vi "Subsystem Sequencer Controller.vi"(8 "error in":errorcluster) -> ()   [LabVIEW 2018]
doc: "This VI executes continuously carrying out the current operation and responding to updates or new operations. It will often contain the timing or control code that is difficult to place directly in TeleOp. This VI generally opens all sensors and motors and isolates the rest of the robot code from knowing how the operations are carried out."
uses:
  <vilib>/Rock Robotics/WPI/Framework/Completion Status.ctl
  Subsystem Sequencer Setpoints.ctl
  Subsystem Sequencer Operations.ctl
  All Commands.ctl
  <vilib>/Rock Robotics/WPI/Solenoid/WPI_SolenoidValue.ctl
  <vilib>/Rock Robotics/WPI/Solenoid/WPI_SolenoidSetEnum.vi
  Wrist/Implementation/Wrist Published Globals.vi
panel:
  in  "In Position":dbl=90.0 format="%#_13g"
  in  "Pickup Position":dbl=-7.0 format="%#_13g"
  out "Value":dbl
  out "Cmd":T1
  in  "Interactive Values":T2
  out "Current\nCmd":string
  in  "Buttons":cluster{"Execute Cmd":bool, "Abort Cmd":bool}
  out "Command Timing":cluster{"Start Time (ms)":u32, "Iterations":i32}
  out "Status":T4
  # "Interactive Command: You may fill in the settings for a command\nand schedule it with the Execute button. You can observe and abort\nany command while fine tuning the code for the controller."
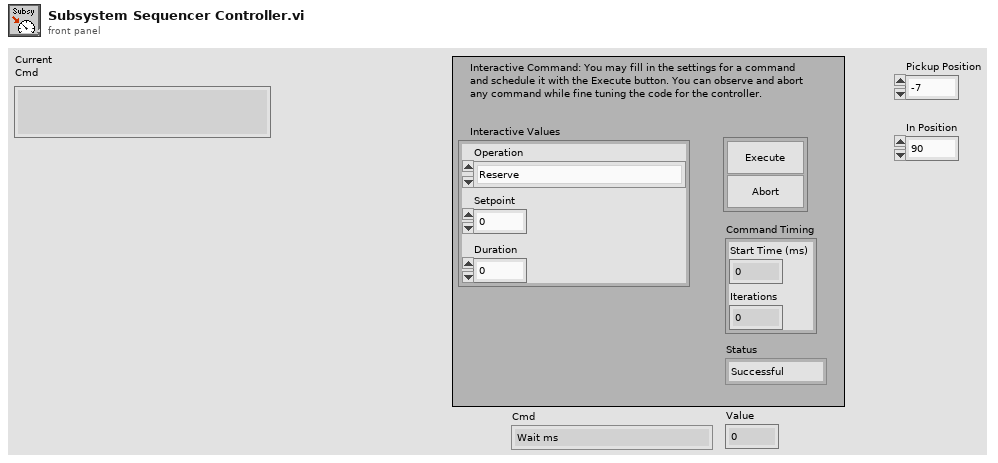
[diagram p1: front panel]
types:
  T1 = typedef "All Commands.ctl" = enum16{"Wait ms", "Drive - Stop Driving", "Drive - Drive Distance Straight", "Elevator - Elevator Stop", "Elevator - Elevator Set Position Wait", "Elevator - Elevator Set Position Start", "Elevator - Wait for Down Fast", "Wrist - Up", "Wrist - Down", "Wrist - Set Position", "Beak - Extend", "Beak - Retract", "Beak - Open", "Beak - Close", "Roller - Off", "Roller - Out", "Roller - In", "Roller - Set Position", "Roller - Wait for Cargo", "Drive - Set Power Straight", "Elevator - Wait Until Stopped", "Leg  - Piston Engage", "Wrist - Set Position Override"}
  T2 = typedef "Subsystem Sequencer Setpoints.ctl" = cluster{"Operation":T3, "Setpoint":dbl, "Duration":dbl}
  T3 = typedef "Subsystem Sequencer Operations.ctl" = enum16{"Reserve", "Read Current", "Run Sequence"}
  T4 = typedef "Completion Status.ctl" = enum16{"Successful", "Aborted", "Incomplete"}
  T5 = typedef "Command Status Info.ctl" = cluster{"Name":string, "Status":T4, "notifier out":T6}
  T6 = typedef "Completion Notifier.ctl" = refnum<notifier>
  T7 = cluster{"Current Command":T2, "Command Timing":cluster{"Start Time (ms)":u32, "Iterations":i32}, "Command Arguments":cluster{"Command Info":T5, "Description":string, "Default Command":T2, "queue out":refnum<queue>, "Subsystem Name":string}}
  T8 = typedef "WPI_SolenoidValue.ctl" = enum16{"Off", "On", "Forward", "Reverse"}
  T9 = typedef "Sequencer Type.ctl" = cluster{"Cmd":T1, "Value":dbl}
  T10 = typedef "WPI_SolenoidDevRef.ctl" = cluster{"DevStatus":errorcluster, "Pneumatics Control Module":u8, "Forward Solenoid Channel":T11, "Reverse Solenoid Channel":T11}
  T11 = typedef "WPI_SolenoidChannel.ctl" = enum8{"Solenoid 0", "Solenoid 1", "Solenoid 2", "Solenoid 3", "Solenoid 4", "Solenoid 5", "Solenoid 6", "Solenoid 7", "Invalid"}
  T12 = typedef "Elevator Telemetry.ctl" = cluster{"Is Moving?":bool, "Setpoint":dbl, "Velocity":dbl, "Position":dbl, "Top Limit":bool, "Bottom Limit":bool, "Applied Output":dbl}
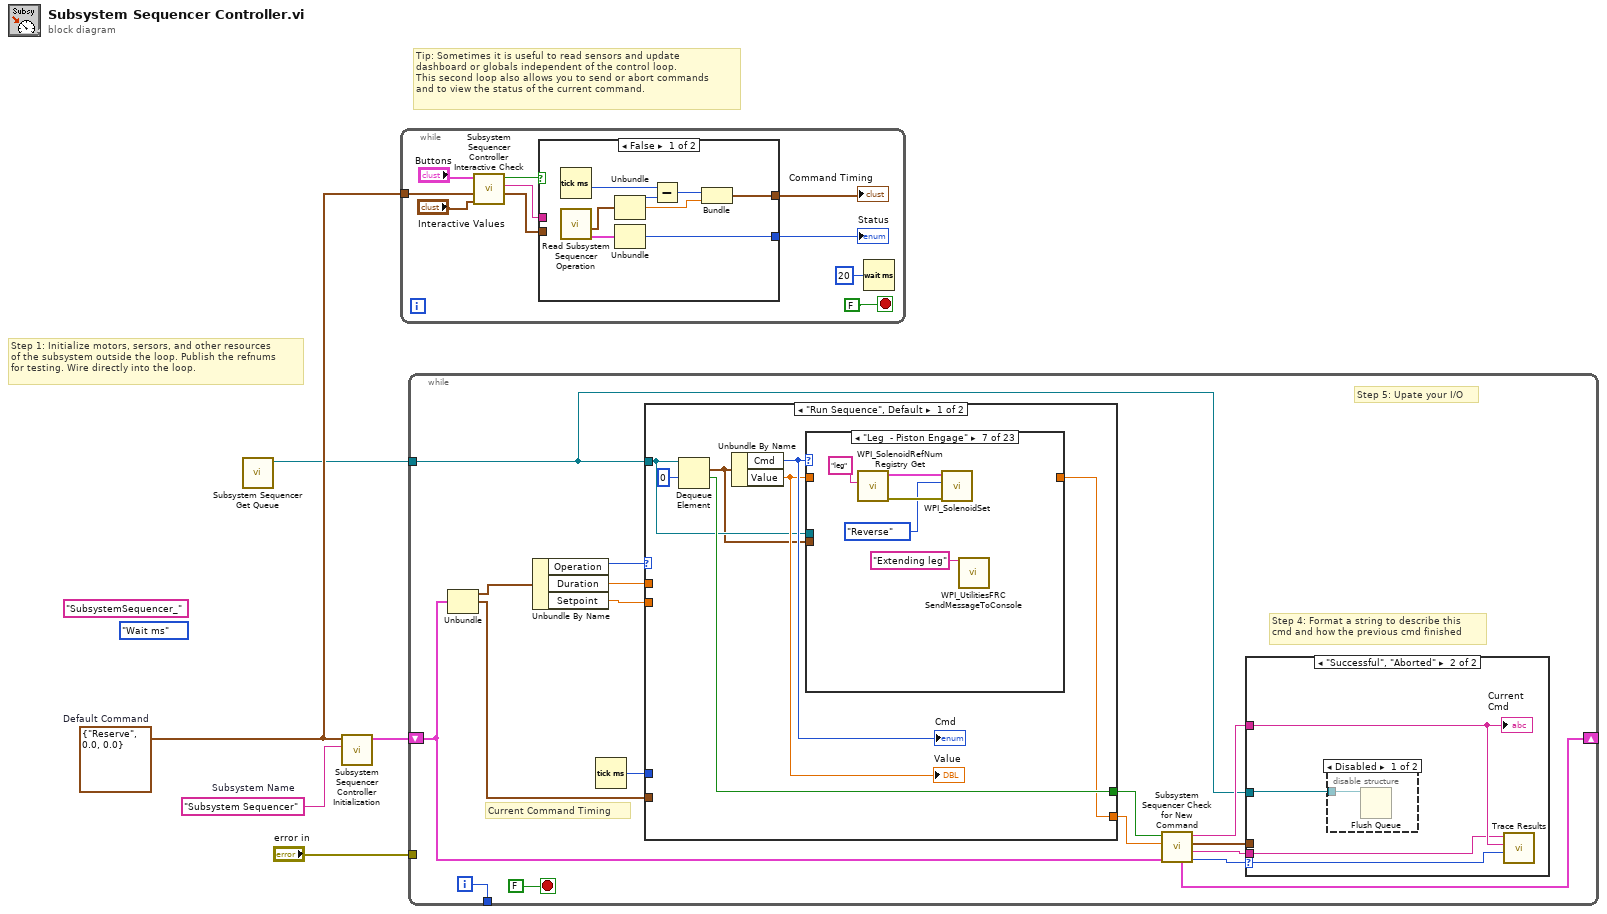
[diagram p0: block diagram]
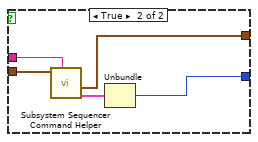
[diagram p2: hidden frame]
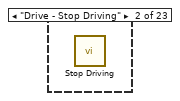
[diagram p6: hidden frame]
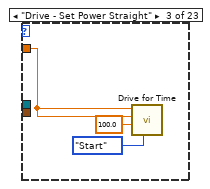
[diagram p7: hidden frame]
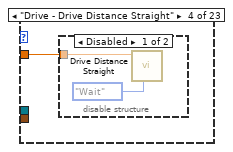
[diagram p8: hidden frame]
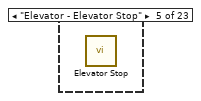
[diagram p10: hidden frame]
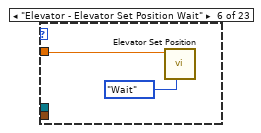
[diagram p11: hidden frame]
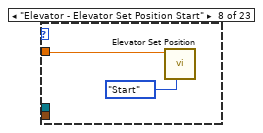
[diagram p12: hidden frame]
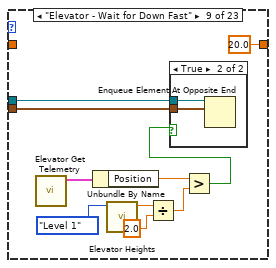
[diagram p13: hidden frame]
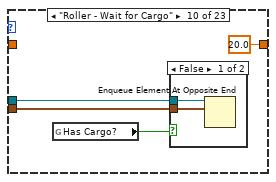
[diagram p15: hidden frame]
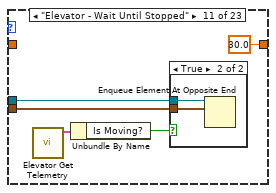
[diagram p17: hidden frame]
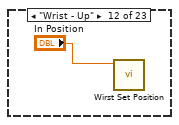
[diagram p19: hidden frame]
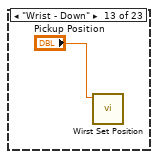
[diagram p20: hidden frame]
diagram:
  (unwired) "SubsystemSequencer_" ("name (unnamed)")
  (unwired) All_Commands."Wait ms" ("Cmd")
  w2 = T2 {"Operation"=enum."Reserve", "Setpoint"=0.0, "Duration"=0.0}  # Default Command
  w3 = "Subsystem Sequencer"  # Subsystem Name
  # "Tip: Sometimes it is useful to read sensors and update\ndashboard or globals independent of the control loop.\nThis second loop also allows you to send or abort commands\nand to view the status of the current command."
  # "Step 1: Initialize motors, sersors, and other resources\nof the subsystem outside the loop. Publish the refnums\nfor testing. Wire directly into the loop."
  n1 = call "Subsystem Sequencer Get Queue.vi"() -> ("queue out"=w1:refnum<queue>)  [unwired: 10 in, 1 out]
  n2 = call "Subsystem Sequencer Controller Initialization.vi"("Subsystem Name"=w3, "Default Command"=w2) -> ("Current Command"=w4:T7)  [unwired: 9 in]
  n3 = while {
    tunnel: w2 -> [w12]
    stop <- FALSE stop-if-true
    n4 = call "Subsystem Sequencer Controller Interactive Check.vi"("Interactive Command in"="Interactive Values", "Default Command"=w12, "Buttons"="Buttons") -> ("Interactive Command out"=w9:T2, "Trace String"=w10:string, "Schedule"=w11:bool)  [unwired: 6 in]
    n5 = case shown="False" w11 {
      tunnel: [w23 w28] -> w8
      tunnel: w9 -> [_ w26]
      tunnel: [w19 w24] -> w7
      tunnel: w10 -> [_ w27]
      frame False {
        n6 = Tick Count (ms)() -> (millisecond timer value=w18:u32)
        n7 = call "Read Subsystem Sequencer Operation.vi"() -> ("Command Info"=w16:T5, "SubSystem Data"=w17:T2)  [unwired: 9 in, 1 out]
        n8 = Unbundle(w17) -> ("Operation"=w22:T3, "Setpoint"=w20:dbl)  [unwired: 1 out]
        n9 = Unbundle(w16) -> ("Status"=w23:T4)  [unwired: 2 out]
        n10 = Subtract(x=w18, y=w22) -> (x-y=w21:u32)
        n11 = Bundle(w21, "Setpoint"=w20) -> (w19:cluster{u32, "Setpoint":dbl})  [unwired: 1 in]
      }
      frame True {
        n12 = call "Subsystem Sequencer Command Helper.vi"("Description"=w27, "SubSystem Data"=w26) -> ("Command Info Out"=w25:T5, "Command Timing"=w24:cluster{"Start Time (ms)":u32, "Iterations":i32})  [unwired: 7 in, 1 out]
        n13 = Unbundle(w25) -> ("Status"=w28:T4)  [unwired: 2 out]
      }
    }
    "Status" <- w8
    "Command Timing" <- w7
    n14 = Wait (ms)(milliseconds to wait=u32 20) -> ()  [unwired: 1 out]
  }
  n15 = while {
    shift-right: [w37] -> _
    shift-left: w4 -> [w30]
    tunnel: [w44] -> _
    tunnel: "error in" -> [_]
    tunnel: w1 -> [w29]
    i -> [w44]
    stop <- FALSE stop-if-true
    # "Step 5: Upate your I/O"
    # "Step 4: Format a string to describe this\ncmd and how the previous cmd finished"
    # "Current Command Timing"
    n16 = Unbundle(w30) -> ("Current Command"=w43:T2, "Command Timing"=w39:cluster{"Start Time (ms)":u32, "Iterations":i32})  [unwired: 1 out]
    n17 = Unbundle By Name(w43) -> ("Operation"=w42:T3, "Duration"=w41:dbl, "Setpoint"=w38:dbl)
    n18 = Tick Count (ms)() -> (millisecond timer value=w40:u32)
    n19 = case shown="\"Run Sequence\", Default" w42 {
      tunnel: [w53 w105] -> w35
      tunnel: [w56 FALSE ("ignore previous (F)")] -> w36
      tunnel: w39 -> [_ _]
      tunnel: w41 -> [_ _]
      tunnel: w40 -> [_ _]
      tunnel: w38 -> [_ _]
      tunnel: w29 -> [w52 _]
      frame "Run Sequence", Default {
        n20 = Dequeue Element(queue=w52, timeout in ms (-1)=0) -> (element=w51:T9, timed out?=w56:bool)  [unwired: 1 in, 2 out]
        n21 = Unbundle By Name(w51) -> ("Cmd"=w55:T1, "Value"=w54:dbl)
        "Cmd" <- w55
        "Value" <- w54
        n22 = case shown="\"Leg  - Piston Engage\"" w55 {
          tunnel: w54 -> [w58 _ w61 w62 _ w66 _ w73 _ _ _ _ _ w101 w102 _ _ _ _ _ w103 _ _]
          tunnel: [w58 _ _ _ _ _ _ _ 20.0 ("Value") 20.0 ("Value") 30.0 ("Value") _ _ _ _ _ _ _ _ _ _ _ _] -> w53
          tunnel: w52 -> [_ _ _ _ _ _ _ _ w83 w89 w96 _ _ _ _ _ _ _ _ _ _ _ _]
          tunnel: w51 -> [_ _ _ _ _ _ _ _ w82 w88 w95 _ _ _ _ _ _ _ _ _ _ _ _]
          frame "Wait ms", Default {
          }
          frame "Drive - Stop Driving" {
            n23 = call "Stop Driving.vi"() -> ()  [unwired: 11 in, 1 out]
          }
          frame "Drive - Set Power Straight" {
            n24 = call "Drive for Time.vi"("Synchronization"=enum16{"Start", "Wait"}."Start", "Seconds"=100.0, "Right Speed"=w61, "Left Speed"=w61) -> ()  [unwired: 6 in, 2 out]
          }
          frame "Drive - Drive Distance Straight" {
            n25 = disable-structure shown="Disabled" {
              disable-tunnel: w62 -> [w64 _]
              frame Disabled {
                n26 = call "Drive Distance Straight.vi"("Synchronication"=enum16{"Start", "Wait"}."Wait", "Distance"=w64) -> ()  [unwired: 9 in, 1 out]
              }
              frame Enabled {
              }
            }
          }
          frame "Elevator - Elevator Stop" {
            n27 = call "Elevator Stop.vi"() -> ()  [unwired: 11 in, 1 out]
          }
          frame "Elevator - Elevator Set Position Wait" {
            n28 = call "Elevator Set Position.vi"("Synchronization"=enum16{"Start", "Wait"}."Wait", "Setpoint"=w66) -> ()  [unwired: 9 in, 1 out]
          }
          frame "Leg  - Piston Engage" {
            n29 = call <vilib>:"WPI_SolenoidRefNum Registry Get.vi"("refnum name"="leg") -> ("error out"=w69:errorcluster, "SolenoidDevRef"=w71:T10)  [unwired: 9 in]
            n30 = call-poly <vilib>:"WPI_SolenoidSet.vi"("error in (no error)"=w69, "Value"=WPI_SolenoidValue."Reverse", "SolenoidDevRef"=w71) -> ()  [unwired: 7 in, 2 out]
            n31 = call <vilib>:"WPI_UtilitiesFRC SendMessageToConsole.vi"("Message"="Extending leg") -> ()  [unwired: 14 in, 1 out]
          }
          frame "Elevator - Elevator Set Position Start" {
            n32 = call "Elevator Set Position.vi"("Synchronization"=enum16{"Start", "Wait"}."Start", "Setpoint"=w73) -> ()  [unwired: 9 in, 1 out]
          }
          frame "Elevator - Wait for Down Fast" {
            n33 = call "Elevator Get Telemetry.vi"() -> ("Telemetry"=w80:T12)  [unwired: 11 in]
            n34 = Unbundle By Name(w80) -> ("Position"=w79:dbl)
            n35 = call "Elevator Heights.vi"("Level"=enum16{"Level 1", "Level 2", "Level 3"}."Level 1") -> ("Height"=w78:dbl)  [unwired: 9 in, 1 out]
            n36 = Divide(x=w78, y=2.0) -> (x/y=w77:dbl)
            n37 = Greater?(x=w79, y=w77) -> (0:w76:bool)
            n38 = case shown="True" w76 {
              tunnel: w83 -> [_ w85]
              tunnel: w82 -> [_ w84]
              frame False {
              }
              frame True {
                n39 = Enqueue Element At Opposite End(queue=w85, element=w84) -> ()  [unwired: 2 in, 3 out]
              }
            }
          }
          frame "Roller - Wait for Cargo" {
            n40 = global read "Wrist Published Globals.vi" "Has Cargo?"() -> (w86:bool)
            n41 = case shown="False" w86 {
              tunnel: w89 -> [w91 _]
              tunnel: w88 -> [w90 _]
              frame False {
                n42 = Enqueue Element At Opposite End(queue=w91, element=w90) -> ()  [unwired: 2 in, 3 out]
              }
              frame True {
              }
            }
          }
          frame "Elevator - Wait Until Stopped" {
            n43 = call "Elevator Get Telemetry.vi"() -> ("Telemetry"=w93:T12)  [unwired: 11 in]
            n44 = Unbundle By Name(w93) -> ("Is Moving?"=w92:bool)
            n45 = case shown="True" w92 {
              tunnel: w96 -> [_ w98]
              tunnel: w95 -> [_ w97]
              frame False {
              }
              frame True {
                n46 = Enqueue Element At Opposite End(queue=w98, element=w97) -> ()  [unwired: 2 in, 3 out]
              }
            }
          }
          frame "Wrist - Up" {
            n47 = call "Wirst Set Position.vi"("Setpoint (Degrees)"="In Position") -> ()  [unwired: 10 in, 1 out]
          }
          frame "Wrist - Down" {
            n48 = call "Wirst Set Position.vi"("Setpoint (Degrees)"="Pickup Position") -> ()  [unwired: 10 in, 1 out]
          }
          frame "Wrist - Set Position Override" {
            n49 = call "Wrist Sensor Set Position Override.vi"("Setpoint"=w101) -> ()  [unwired: 10 in, 1 out]
          }
          frame "Wrist - Set Position" {
            n50 = call "Wirst Set Position.vi"("Setpoint (Degrees)"=w102) -> ()  [unwired: 10 in, 1 out]
          }
          frame "Beak - Extend" {
            n51 = call "Beak Extend.vi"() -> ()  [unwired: 11 in, 1 out]
          }
          frame "Beak - Retract" {
            n52 = call "Beak Retract.vi"() -> ()  [unwired: 11 in, 1 out]
          }
          frame "Beak - Open" {
            n53 = call "Beak Open.vi"() -> ()  [unwired: 11 in, 1 out]
          }
          frame "Beak - Close" {
            n54 = call "Beak Close.vi"() -> ()  [unwired: 11 in, 1 out]
          }
          frame "Roller - Off" {
            n55 = call "Rollers Off.vi"() -> ()  [unwired: 11 in, 1 out]
          }
          frame "Roller - Set Position" {
            n56 = call "Set Roller Speed.vi"("Setpoint"=w103) -> ()  [unwired: 10 in, 1 out]
          }
          frame "Roller - Out" {
            n57 = call "Rollers Out.vi"() -> ()  [unwired: 11 in, 1 out]
          }
          frame "Roller - In" {
            n58 = call "Rollers In.vi"() -> ()  [unwired: 11 in, 1 out]
          }
        }
      }
      frame "Reserve" {
        w105 = 100.0  # Infinite
        # "For debugging the sensor"
      }
    }
    n59 = call "Subsystem Sequencer Check for New Command.vi"("Current Command"=w30, "Wait time (ms)"=w35, "Finished?"=w36) -> ("Completion"=w31:T4, "Subsystem Name"=w32:string, "Current Command"=w33:T2, "Initial Trace String"=w34:string, "NextCommand"=w37:T7)  [unwired: 4 in]
    n60 = case shown="\"Successful\", \"Aborted\"" w31 {
      selector: w31 -> [_ w49]
      tunnel: w34 -> [_ w48]
      tunnel: w33 -> [_ _]
      tunnel: w32 -> [_ w47]
      tunnel: w29 -> [_ w46]
      frame "Incomplete", Default {
        # "Continuing current command"
      }
      frame "Successful", "Aborted" {
        # "Report and setup for next command"
        n61 = disable-structure shown="Disabled" {
          disable-tunnel: w46 -> [w50 _]
          frame Disabled {
            n62 = Flush Queue(queue=w50) -> ()  [unwired: 1 in, 3 out]
          }
          frame Enabled {
          }
        }
        n63 = call <vilib>:"Trace Results.vi"("Status of previous command"=w49, "Description"=w48, "Subsystem"=w47) -> ()  [unwired: 9 in]
        "Current\nCmd" <- w48
      }
    }
  }
